vi "getFrameSize.vi"(8 "error":errorcluster, 11 "connection ID":refnum<k5>) -> (0 "error out":errorcluster, 1 "FrameSize":i32, 3 "connection ID out":refnum<k5>)   [LabVIEW 2016, in "AMC_VIs.lvlib"]
doc: "This function reads the frame size of the RES chain \nInputs:\n -- connection string (from connect_TCP.vi)\n\n\nOutputs:\n -- connection ID out\n -- Frame Size"
uses:
  AMC_VIs.lvlib
panel:
  out "JSON-response":string="{\"jsonrpc\":\"2.0\",\"method\":\"\",\"params\":[5,1.245,true,\"name\"],\"id\":\"1\"}"
  out "JSON request":string
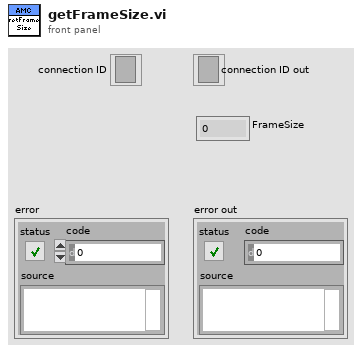
[diagram p1: front panel]
types:
  T1 = cluster{"jsonrpc":string, "method":string, "params":i32[], "id":string, "api":string}
  T2 = cluster{"jsonrpc":string, "result":i32[], "id":string}
  T3 = enum16{"Standard", "Buffered", "CRLF", "Immediate"}
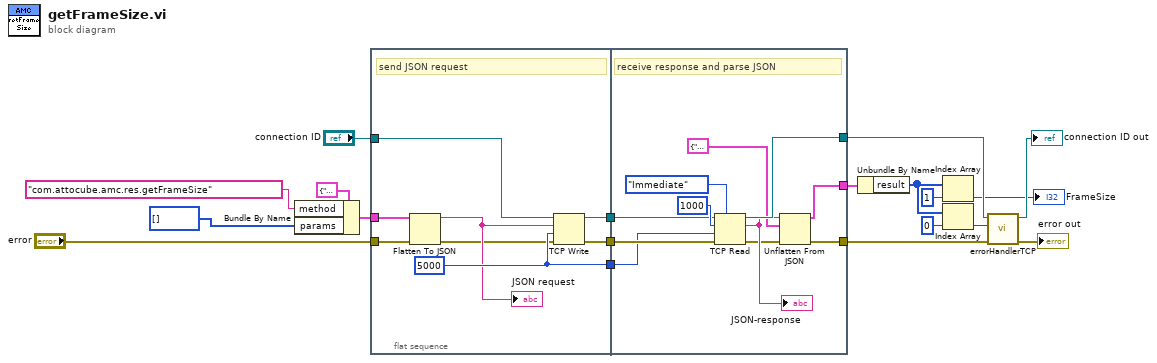
[diagram p0: block diagram]
diagram:
  n1 = Bundle By Name(cluster=T1 {"jsonrpc"="2.0", "method"="com.attocube.amc.res.setRESReadOutFreq", "params"=[0, 2712], "id"="1", "api"="2"} ("InputParams 2"), "method"="com.attocube.amc.res.getFrameSize", "params"=i32[] []) -> (w12:T1)
  n2 = flat-sequence {
    tunnel: "connection ID" -> [w27]
    tunnel: [w25] -> w19
    tunnel: [w26] -> w18
    tunnel: "error" -> [w21]
    tunnel: [w24] -> w17
    tunnel: w12 -> [w23]
    tunnel: [w34] -> w4
    tunnel: w19 -> [w36]
    tunnel: w18 -> [w35]
    tunnel: [w30] -> w7
    tunnel: w17 -> [w33]
    tunnel: [w29] -> w11
    frame #0 {
      w24 = 5000 ("timeout ms (25000)")
      # "send JSON request"
      n3 = Flatten To JSON(anything=w23, error in (no error)=w21) -> (JSON string=w22:string, 11:w20:errorcluster)  [unwired: 1 in]
      "JSON request" <- w22
      n4 = TCP Write(connection ID=w27, data in=w22, error in (no error)=w20, 9:w24) -> (connection ID out=w25:refnum<k5>, error out=w26:errorcluster)  [unwired: 1 out]
    }
    frame #1 {
      # "receive response and parse JSON"
      n5 = TCP Read(connection ID=w36, bytes to read=1000, error in (no error)=w35, 7:T3."Immediate" ("mode (standard)"), 9:w33) -> (connection ID out=w34:refnum<k5>, data out=w32:string, error out=w31:errorcluster)
      "JSON-response" <- w32
      n6 = Unflatten From JSON(JSON string=w32, type and defaults=T2 {"jsonrpc"="2.0", "result"=[0, 2712], "id"="1"} ("InputParams 2"), error in (no error)=w31) -> (value=w29:T2, error out=w30:errorcluster)  [unwired: 4 in]
    }
  }
  n7 = Unbundle By Name(w11) -> ("result"=w8:i32[])
  n8 = Index Array(array=w8, index=1) -> (element=→"FrameSize":i32)
  n9 = Index Array(array=w8, index=0) -> (element=w6:i32)
  n10 = call "errorHandlerTCP.vi"("error in"=w7, "error number"=w6, "connection ID"=w4) -> ("error out"=→"error out":errorcluster, "connection ID"=→"connection ID out":refnum<k5>)  [unwired: 7 in]
